vi "example_microFPGA_lasers.vi"() -> ()   [LabVIEW 2021]
panel:
  in  "laser channel":u16(ring)=1 items=["channel No 0", "channel No 1", "channel No 2", "channel No 3", "channel No 4", "channel No 5", "channel No 6", "channel No 7"]
  out "Laser_duration_READ":u32(slide)=9 max=65535 step=1 scale=0.0..65535.0 scale format="%u us"
  out "Laser_sequence_READ":bool[](array[boolean])=[FALSE, TRUE, FALSE, TRUE, FALSE, TRUE, FALSE, TRUE, FALSE, TRUE, FALSE, TRUE, FALSE, TRUE, FALSE, TRUE, FALSE, FALSE, FALSE, FALSE, FALSE, FALSE, FALSE, FALSE, FALSE, FALSE, FALSE, FALSE, FALSE, FALSE, FALSE, FALSE]
  out "Laser_mode_READ":u16(ring)=4 items=["OFF", "ON", "RISING", "FALLING", "FOLLOW"]
  in  "write or read":u16(ring)=1 items=["read", "write"]
  out "value write confirm 3":bool
  out "value write confirm 2":bool
  out "value write confirm":bool
  out "Version":u16=3
  in  "Laser_mode_WRITE":u16(ring)=4 items=["OFF", "ON", "RISING", "FALLING", "FOLLOW"]
  in  "Laser_sequence_WRITE":bool[](array[boolean])=[FALSE, TRUE, FALSE, TRUE, FALSE, TRUE, FALSE, TRUE, FALSE, TRUE, FALSE, TRUE, FALSE, TRUE, FALSE, TRUE]
  in  "Laser_duration_WRITE":u32(slide)=9 max=65535 step=1 scale=0.0..65535.0 scale format="%u us"
  in  "close Application":bool=TRUE
  in  "send parameters":bool
  # "Laser control"
  # "0"
  # "7"
  # "15"
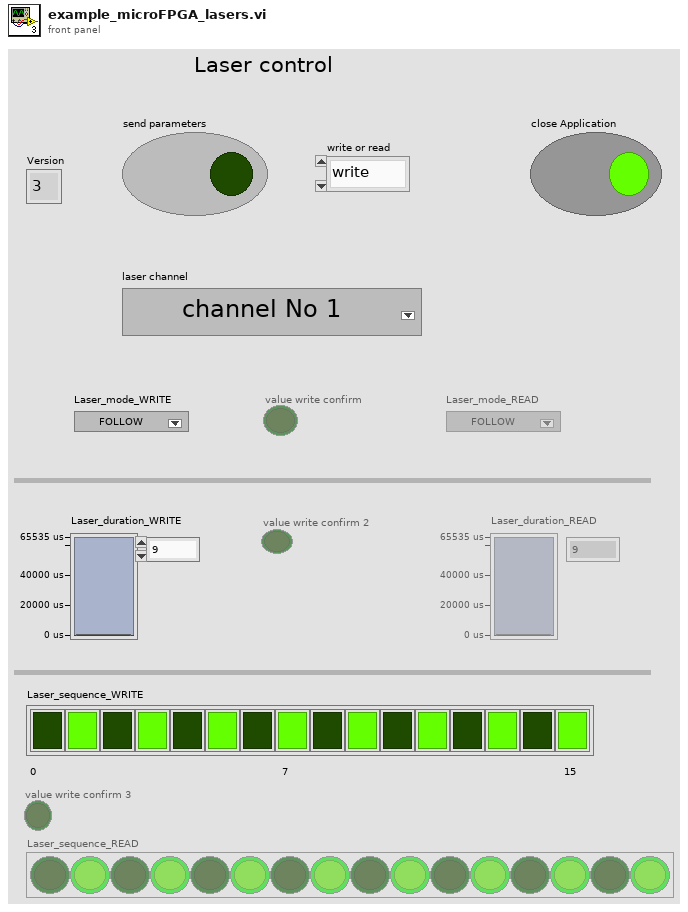
[diagram p1: front panel]
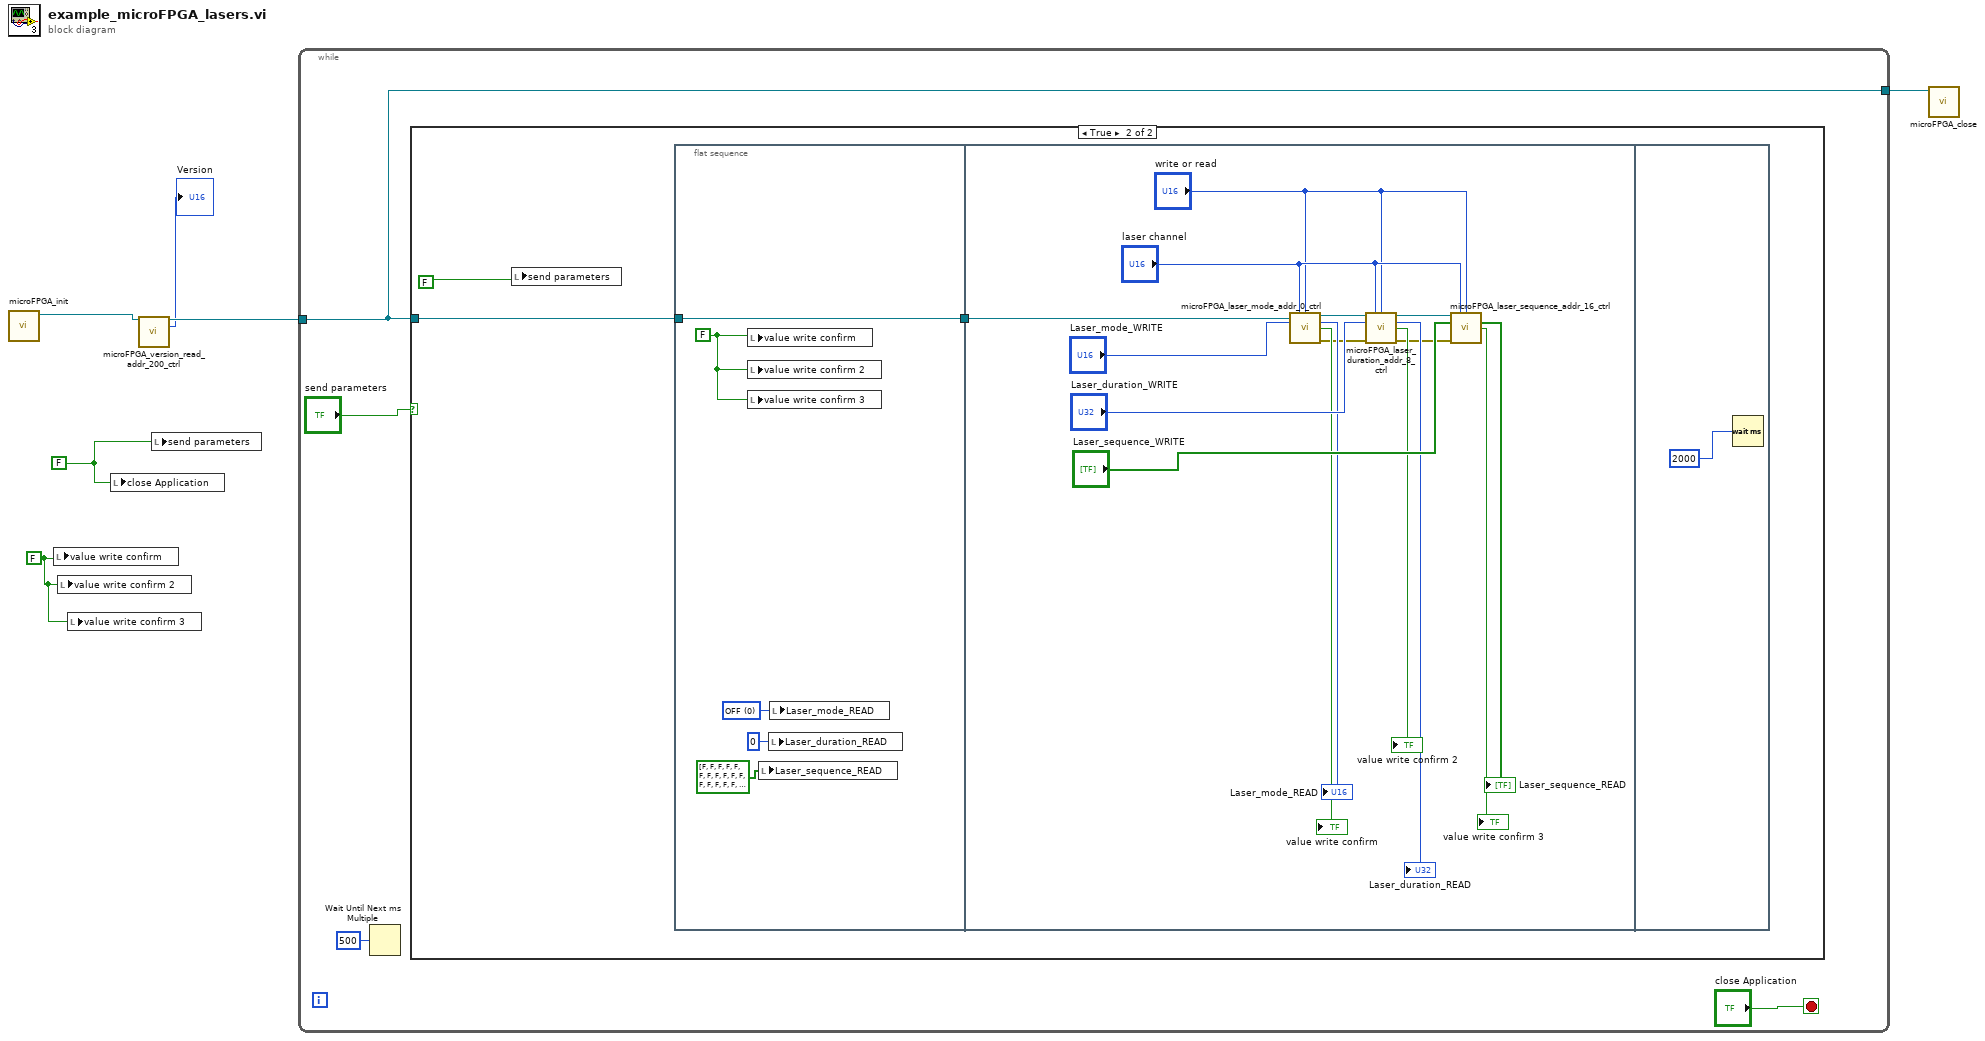
[diagram p0: block diagram]
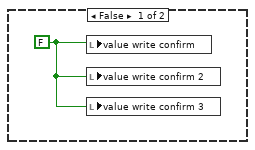
[diagram p2: hidden frame]
diagram:
  w1 = FALSE ("write")
  w6 = FALSE ("write")
  n1 = call "microFPGA_init.vi"() -> ("VISA resource name out"=w4:refnum<visa-resource-name>)  [unwired: 10 in, 1 out]
  n2 = local write "value write confirm"(w1) -> ()
  n3 = local write "value write confirm 2"(w1) -> ()
  n4 = local write "value write confirm 3"(w1) -> ()
  n5 = local write "close Application"(w6) -> ()
  n6 = call "microFPGA_version_read_addr_200_ctrl.vi"("VISA resource name"=w4) -> ("VISA resource name 2"=w3:refnum<visa-resource-name>, "Version"=→"Version":u16)  [unwired: 12 in, 1 out]
  n7 = local write "send parameters"(w6) -> ()
  n8 = while {
    tunnel: w3 -> [w7]
    tunnel: [w7] -> w5
    stop <- "close Application" stop-if-true
    n9 = Wait Until Next ms Multiple(millisecond multiple=u32 500) -> ()  [unwired: 1 out]
    n10 = case shown="True" "send parameters" {
      tunnel: w7 -> [_ w13]
      frame False {
        w11 = FALSE ("value write confirm")
        n11 = local write "value write confirm"(w11) -> ()
        n12 = local write "value write confirm 2"(w11) -> ()
        n13 = local write "value write confirm 3"(w11) -> ()
      }
      frame True {
        n14 = local write "send parameters"(FALSE ("write")) -> ()
        n15 = flat-sequence {
          tunnel: w13 -> [w19]
          tunnel: [w19] -> w12
          tunnel: w12 -> [w35]
          frame #0 {
            w16 = u16 0 items=["OFF", "ON", "RISING", "FALLING", "CAMERA"] ("Laser_mode_READ")
            w15 = FALSE ("value write confirm")
            n16 = local write "value write confirm"(w15) -> ()
            n17 = local write "value write confirm 2"(w15) -> ()
            n18 = local write "value write confirm 3"(w15) -> ()
            n19 = local write "Laser_sequence_READ"(bool[] [FALSE, FALSE, FALSE, FALSE, FALSE, FALSE, FALSE, FALSE, FALSE, FALSE, FALSE, FALSE, FALSE, FALSE, FALSE, FALSE, FALSE, FALSE, FALSE, FALSE, FALSE, FALSE, FALSE, FALSE, FALSE, FALSE, FALSE, FALSE, FALSE, FALSE, FALSE, FALSE] ("Laser_sequence_READ")) -> ()
            n20 = local write "Laser_duration_READ"(u32 0 ("Laser_duration_READ")) -> ()
            n21 = local write "Laser_mode_READ"(w16) -> ()
          }
          frame #1 {
            n22 = call "microFPGA_laser_mode_addr_0_ctrl.vi"("VISA resource name"=w35, "laser channel"="laser channel", "write or read"="write or read", "Laser_mode_WRITE"="Laser_mode_WRITE") -> ("VISA resource name 2"=w33:refnum<visa-resource-name>, "Laser_mode_READ"=→"Laser_mode_READ":u16, "value write confirm"=→"value write confirm":bool, "error out"=w21:errorcluster)  [unwired: 7 in, 1 out]
            n23 = call "microFPGA_laser_duration_addr_8_ctrl.vi"("VISA resource name"=w33, "laser channel"="laser channel", "write or read"="write or read", "Laser_duration_WRITE"="Laser_duration_WRITE", "error in (no error)"=w21) -> ("VISA resource name 2"=w30:refnum<visa-resource-name>, "Laser_duration_READ"=→"Laser_duration_READ":u32, "value write confirm"=→"value write confirm 2":bool, "error out"=w22:errorcluster)  [unwired: 6 in, 1 out]
            n24 = call "microFPGA_laser_sequence_addr_16_ctrl.vi"("VISA resource name"=w30, "laser channel"="laser channel", "write or read"="write or read", "Laser_sequence_WRITE"="Laser_sequence_WRITE", "error in (no error)"=w22) -> ("Laser_sequence_READ"=→"Laser_sequence_READ":bool[], "value write confirm"=→"value write confirm 3":bool)  [unwired: 6 in, 3 out]
          }
          frame #2 {
            n25 = Wait (ms)(milliseconds to wait=u32 2000 ("milliseconds to RUN")) -> ()  [unwired: 1 out]
          }
        }
      }
    }
  }
  n26 = call "microFPGA_close.vi"("VISA resource name"=w5) -> ()  [unwired: 11 in]
